vi "Acc_pipeline_phase1_2.vi"(9 "path 2":path=path "C:/Users/TIDAS/OneDrive - University of Gothenburg/TietzeLab/Autodata_Exp/testdata", 11 "module path":path=path "C:/Users/TIDAS/OneDrive - University of Gothenburg/TietzeLab/Pyhton scripts_labview/Script for Stage II_labview/Save_data.py") -> ()   [LabVIEW 2021]
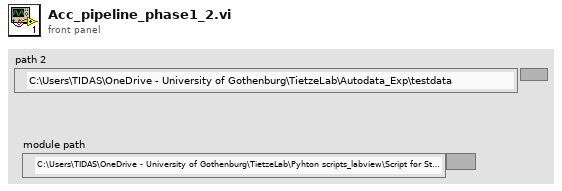
[diagram p1: front panel]
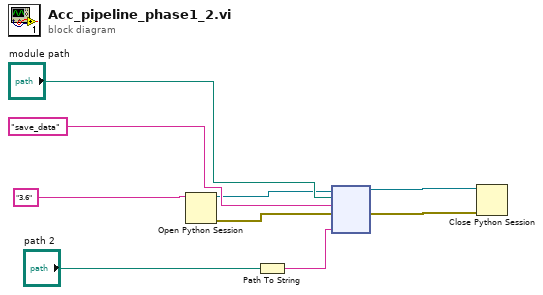
[diagram p0: block diagram]
diagram:
  n1 = Open Python Session(python version="3.6" ("Python version")) -> (session out=w4:refnum<k35>, error out=w3:errorcluster)  [unwired: 2 in]
  n2 = Path To String(path="path 2") -> (string=w7:string)
  n3 = node(w4, "module path", "save_data" ("function name"), w3, w7) -> (w2:refnum<k35>, w1:errorcluster)  [unwired: 3 in, 2 out]
  n4 = Close Python Session(session in=w2, error in=w1) -> ()  [unwired: 1 out]
